vi "Truncate.vi"(1 "Number of Digits":i16=1, 2 "Number":dbl=1.4939637826961771 format="%#_8g") -> (0 "Truncated Number":dbl format="%#_8g")   [LabVIEW 2014]
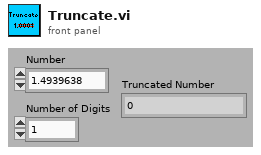
[diagram p1: front panel]
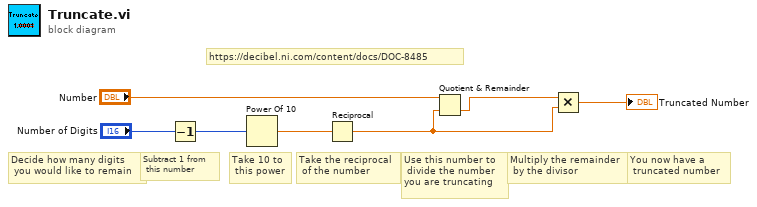
[diagram p0: block diagram]
diagram:
  # "https://decibel.ni.com/content/docs/DOC-8485"
  # "You now have a\n truncated number"
  # "Multiply the remainder\n by the divisor"
  # "Use this number to\n divide the number \nyou are truncating"
  # "Take the reciprocal\n of the number"
  # "Take 10 to\n this power"
  # "Subtract 1 from\n this number"
  # "Decide how many digits\n you would like to remain"
  n1 = Decrement(x="Number of Digits") -> (x-1=w1:i16)
  n2 = Power Of 10(x=w1) -> (10^x=w4:dbl)
  n3 = Reciprocal(x=w4) -> (1/x=w3:dbl)
  n4 = Quotient & Remainder(x="Number", y=w3) -> (floor(x/y)=w6:dbl)  [unwired: 1 out]
  n5 = Multiply(x=w6, y=w3) -> (x*y=→"Truncated Number":dbl)
